vi "SetClassCtrl.vi"(8 "error in (no error)":errorcluster caption="entrée d'erreur (pas d'erreur)", 10 "ClassCtrlRef":refnum<vi>, 11 "OR77200 en entrée":refnum<class "OR77200.lvclass"> caption="DNL_LabVIEW Object in") -> (0 "error out":errorcluster caption="sortie d'erreur", 3 "OR77200 en sortie":refnum<class "OR77200.lvclass"> caption="DNL_LabVIEW Object out")   [LabVIEW 2012, in "OR77200.lvclass"]
uses:
  OR77200.lvclass
  BaseDevice/BaseDevice.lvclass
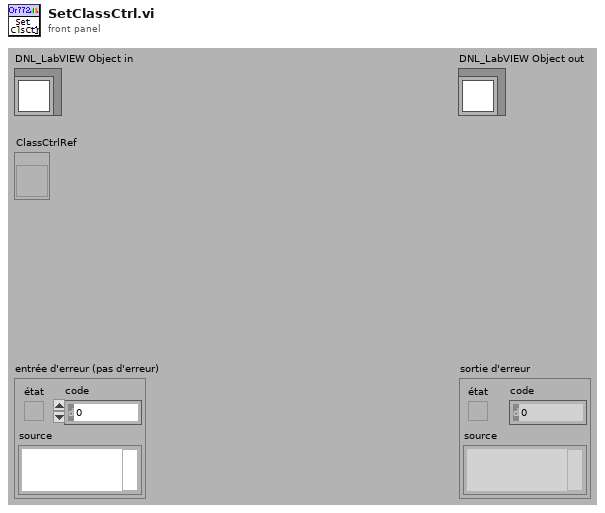
[diagram p1: front panel]
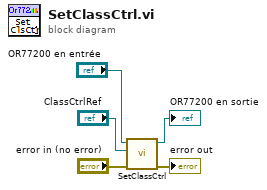
[diagram p0: block diagram]
diagram:
  n1 = call-parent "SetClassCtrl.vi"("error in (no error)"="error in (no error)", "ClassCtrlRef"="ClassCtrlRef", "BaseDevice en entrée"="OR77200 en entrée") -> ("error out"=→"error out":errorcluster, "BaseDevice en sortie"=→"OR77200 en sortie":refnum<class "OR77200.lvclass">)  [unwired: 7 in]
